vi "dsdll_output_status.vi"(8 "error in":errorcluster, 11 "dsdll instance in":T2={"dsdll path"=path "E:/LVprog/DirectSoundDLL/dsdll.dll", "dsdll handle"=[], "output devices"=[], "capture devices"=[]}) -> (0 "error out":errorcluster, 1 "cursor position [%]":i32, 2 "output buffer exists?":bool, 3 "dsdll instance out":T2, 4 "playback cursor":u32, 5 "format":T1, 6 "buffer length":u32)   [LabVIEW 2013, in "dsdll.lvlib"]
doc: "Call to get status of playback buffer. This VI changes nothing in the DSDLL instance so it can be called from a different thread/process and the 'dsdll instance out' is optional."
uses:
  dsdll.lvlib
  dsdll_instance.ctl
  dsdll_device_record.ctl
  dsdll_sample_format.ctl
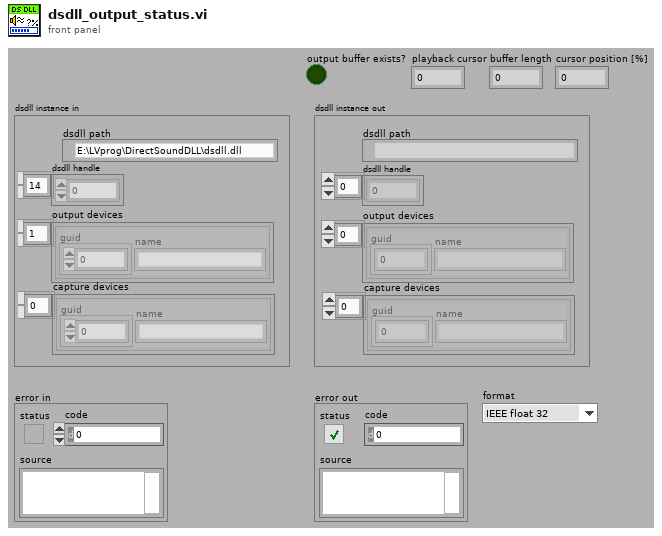
[diagram p1: front panel]
types:
  T1 = typedef "dsdll.lvlib/dsdll_sample_format.ctl" = enum16{"IEEE float 32", "PCM 16 bit"}
  T2 = typedef "dsdll.lvlib/dsdll_instance.ctl" = cluster{"dsdll path":path, "dsdll handle":u8[], "output devices":T3[], "capture devices":T3[]}
  T3 = typedef "dsdll.lvlib/dsdll_device_record.ctl" = cluster{"guid":u8[], "name":string}
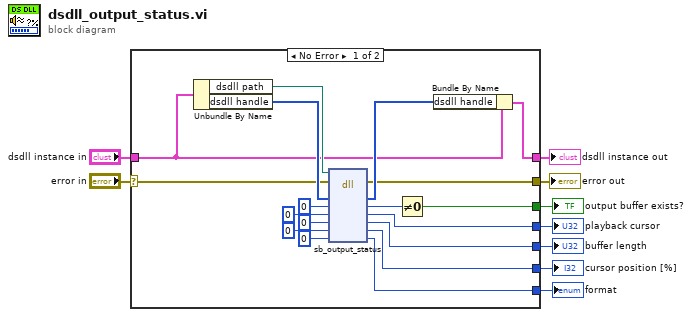
[diagram p0: block diagram]
diagram:
  n1 = case shown="No Error" "error in" {
    selector: "error in" -> [w23 w28]
    tunnel: "dsdll instance in" -> [w13 w29]
    tunnel: [w12 w28] -> w8
    tunnel: [w24 w29] -> w9
    tunnel: [w17 _] -> w5
    tunnel: [w16 _] -> w4
    tunnel: [w15 _] -> w3
    tunnel: [w14 _] -> w2
    tunnel: [w10 _] -> w1
    frame No Error {
      n2 = Unbundle By Name(w13) -> ("dsdll path"=w27:path, "dsdll handle"=w26:u8[])
      n3 = dll-call lib="dsdll.dll" fn="sb_output_status" ("sb_get_handle_size()")(path in=w27, error in=w23, "handle"=w26, "status"=0, "smpl_pos"=u32 0, "smpl_count"=u32 0, "proc"=0, "format"=u16 0) -> (error out=w12:errorcluster, "handle"=w25:u8[], "status"=w18:i32, "smpl_pos"=w16:u32, "smpl_count"=w15:u32, "proc"=w14:i32, "format"=w10:u16)  [unwired: 2 in, 1 out]
      n4 = Not Equal To 0?(x=w18) -> (x != 0?=w17:bool)
      n5 = Bundle By Name(cluster=w13, "dsdll handle"=w25) -> (w24:T2)
    }
    frame Error {
    }
  }
  "error out" <- w8
  "dsdll instance out" <- w9
  "output buffer exists?" <- w5
  "playback cursor" <- w4
  "buffer length" <- w3
  "cursor position [%]" <- w2
  "format" <- w1
